vi "Pockels Cal_Update core.vi"(7 "Create new?":bool, 9 "New cal section (empty objectives removed)":string[][](array[string])=[["Cal Wavelength", "", "", "", "", "", ""], ["920", "", "", "", "", "", ""], ["Cal subset indexes", "", "", "", "", "", ""], ["0", "15", "", "", "", "", ""], ["Cal data", "", "", "", "", "", ""], ["Pockels V", "No objective", "Olympus 60X", "Empty new", "Olympus 20X", "Brand new", "Nikon 25X"], ["0", "11", "1", "", "1000", "100", ""], ["0.111", "22", "2", "", "2000", "200", ""], ["0.222", "33", "3", "", "3000", "300", ""], ["0.333", "44", "4", "", "", "400", ""], ["0.444", "55", "5", "", "", "500", ""], ["0.5", "66", "6", "", "", "", ""], ["0.6", "77", "7", "", "", "", ""], ["0.7", "88", "8", "", "", "", ""], ["0.8", "99", "9", "", "", "", ""], ["0.9", "00", "0", "", "", "", ""], ["1", "11", "1", "", "", "", ""], ["1.1", "22", "2", "", "", "", ""], ["1.2", "33", "3", "", "", "", ""], ["1.3", "44", "4", "", "", "", ""], ["1.4", "55", "5", "", "", "", ""], ["1.5", "66", "6", "", "", "", ""], ["1.6", "77", "7", "", "", "", ""], ["1.7", "88", "8", "", "", "", ""], ["1.8", "99", "9", "", "", "", ""], ["1.9", "00", "0", "", "", "", ""], ["2", "11", "1", "900", "9000", "", ""]], 11 "Loaded cal file":string[][](array[string])=[["Cal Wavelength", "", "", "", "", ""], ["800", "", "", "", "", ""], ["Cal subset indexes", "", "", "", "", ""], ["0", "15", "", "", "", ""], ["Cal data", "", "", "", "", ""], ["Pockels V", "No objective", "Olympus 20X", "Nikon 25X", "Olympus 40X", "Olympus 60X"], ["0", "1.9", "", "", "", ""], ["0.1", "3.7", "", "", "", ""], ["0.2", "8.2", "", "", "", ""], ["0.3", "15.4", "", "", "", ""], ["0.4", "24.5", "", "", "", ""], ["0.5", "35.5", "", "", "", ""], ["0.6", "47.8", "", "", "", ""], ["0.7", "61.3", "", "", "", ""], ["0.8", "73.4", "", "", "", ""], ["0.9", "90", "", "", "", ""], ["1", "104", "", "", "", ""], ["1.1", "116", "", "", "", ""], ["1.2", "128", "", "", "", ""], ["1.3", "138", "", "", "", ""], ["1.4", "148", "", "", "", ""], ["1.5", "154", "", "", "", ""], ["1.6", "157", "", "", "", ""], ["1.7", "155", "", "", "", ""], ["1.8", "154", "", "", "", ""], ["1.9", "154", "", "", "", ""], ["2", "154", "", "", "", ""], ["", "", "", "", "", ""], ["Cal Wavelength", "", "", "", "", ""], ["920", "", "", "", "", ""], ["Cal subset indexes", "", "", "", "", ""], ["0", "15", "", "", "", ""], ["Cal data", "", "", "", "", ""], ["Pockels V", "No objective", "Olympus 20X", "Nikon 25X", "Olympus 40X", "Olympus 60X"], ["0", "1.9", "1", "2", "", ""], ["0.1", "3.7", "1", "2", "", ""], ["0.2", "8.2", "1", "2", "", ""], ["0.3", "15.4", "1", "2", "", ""], ["0.4", "24.5", "1", "2", "", ""], ["0.5", "35.5", "1", "", "", ""], ["0.6", "47.8", "1", "", "", ""], ["0.7", "61.3", "1", "", "", ""], ["0.8", "73.4", "", "", "", ""], ["0.9", "90", "", "", "", ""], ["1", "104", "", "", "", ""], ["1.1", "116", "", "", "", ""], ["1.2", "128", "", "", "", ""], ["1.3", "138", "", "", "", ""], ["1.4", "148", "", "", "", ""], ["1.5", "154", "", "", "", ""], ["1.6", "157", "", "", "", ""], ["1.7", "155", "", "", "", ""], ["1.8", "154", "", "", "", ""], ["1.9", "154", "1", "2", "", ""], ["2", "154", "1", "2", "", ""], ["", "", "", "", "", ""]]) -> (2 "Cal file strings":string[][](array[string]))   [LabVIEW 2020]
panel:
  out "Current wavelength":dbl
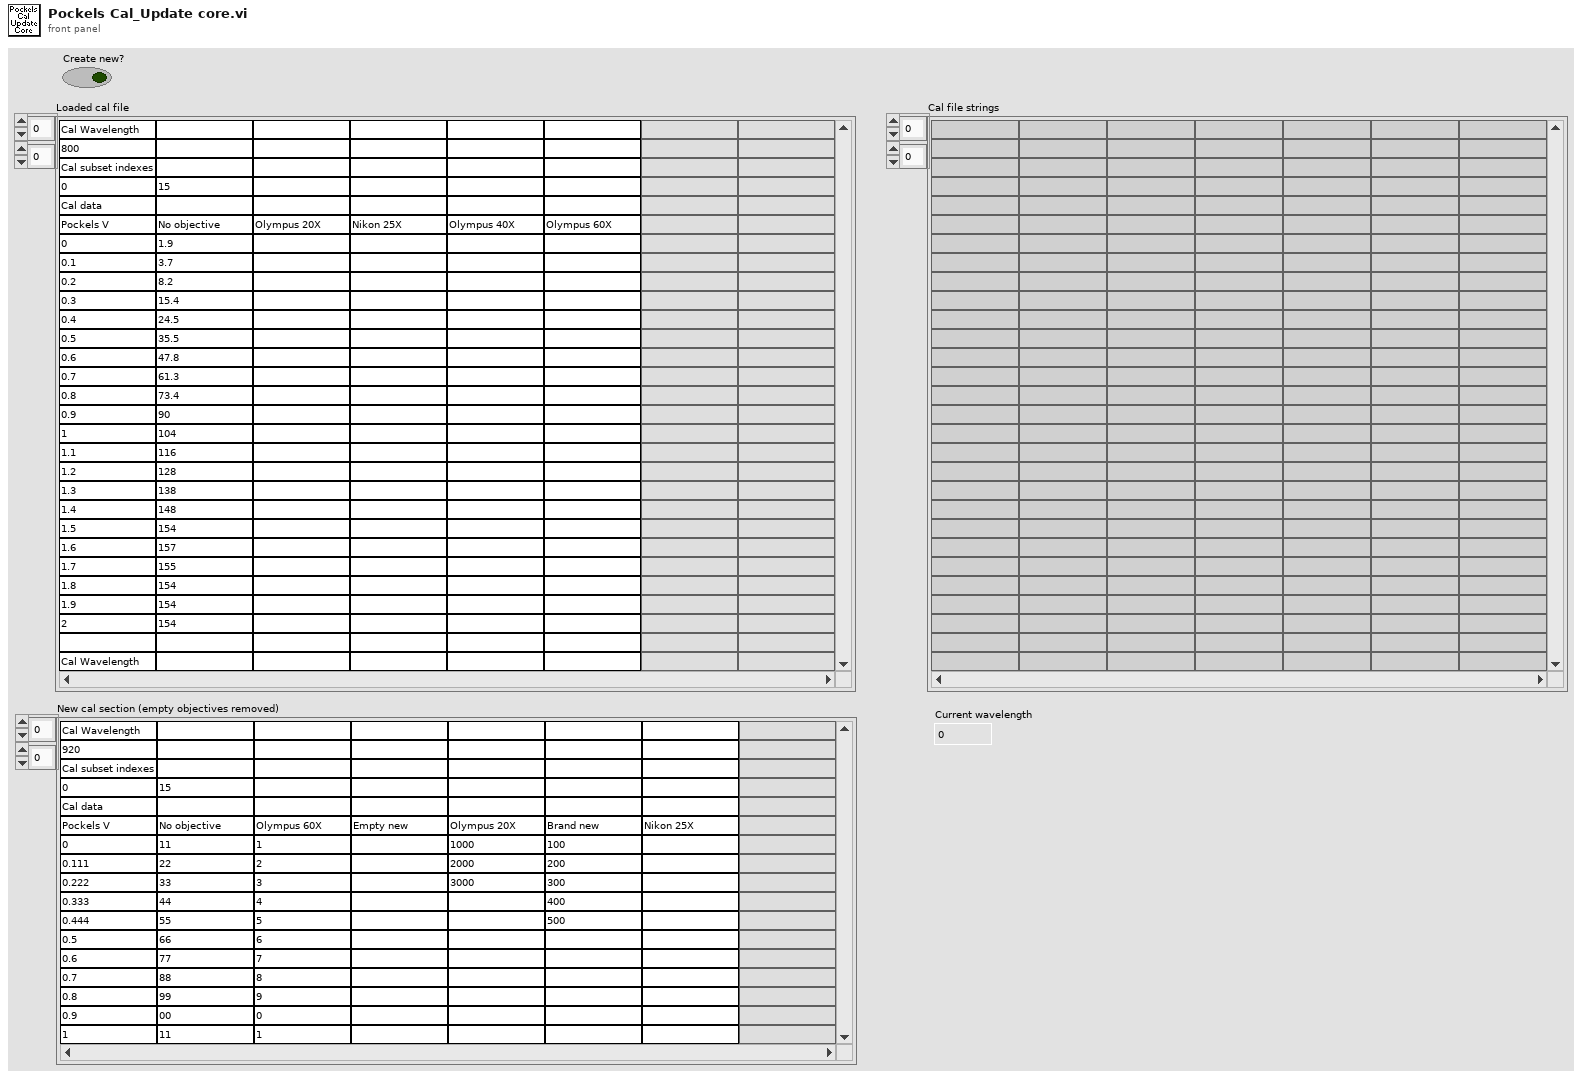
[diagram p1: front panel]
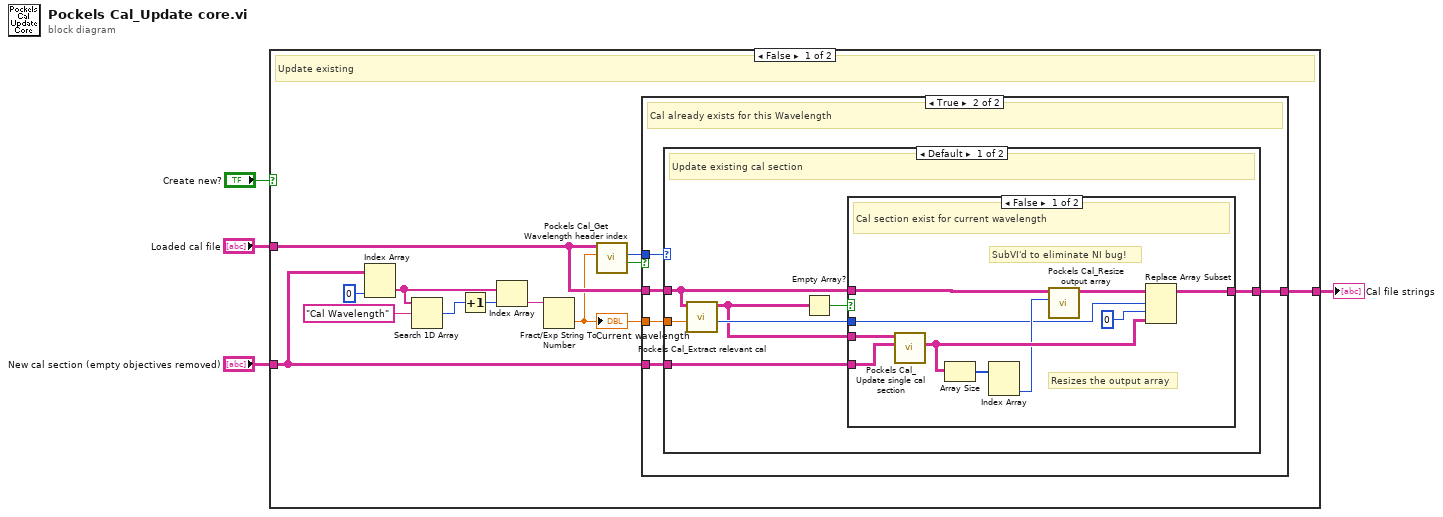
[diagram p0: block diagram]
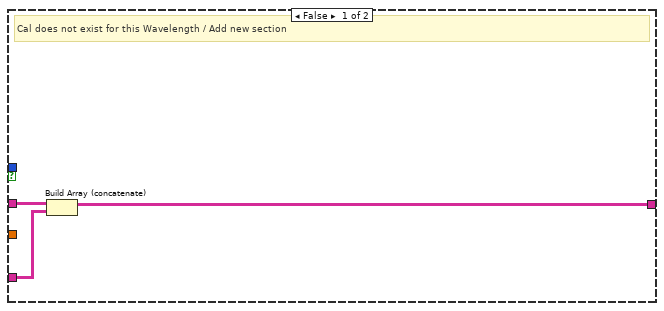
[diagram p2: hidden frame]
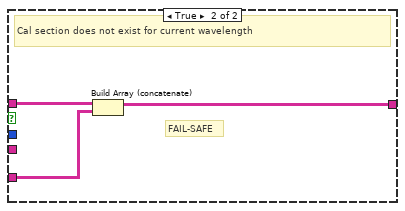
[diagram p3: hidden frame]
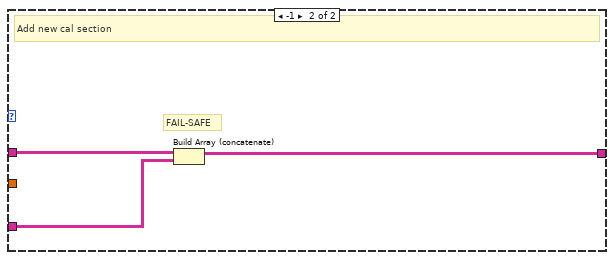
[diagram p4: hidden frame]
diagram:
  n1 = case shown="False" "Create new?" {
    tunnel: [w11 w48] -> w4
    tunnel: "Loaded cal file" -> [w7 _]
    tunnel: "New cal section (empty objectives removed)" -> [w6 w48]
    frame False {
      # "Update existing"
      n2 = Index Array(array=w6, index (col)=0 ("disabled index (col)")) -> (element=w14:string[])  [unwired: 1 in]
      n3 = Search 1D Array(1D array=w14, element="Cal Wavelength") -> (index of element=w15:i32)  [unwired: 1 in]
      n4 = Increment(x=w15) -> (x+1=w12:i32)
      n5 = Index Array(array=w14, index=w12) -> (element=w13:string)
      n6 = Fract/Exp String To Number(string=w13) -> (number=w5:dbl)  [unwired: 3 in, 1 out]
      "Current wavelength" <- w5
      n7 = call "Pockels Cal_Get Wavelength header index.vi"("Waveform"=w5, "Loaded cal file"=w7) -> ("Cal already exists for this wavelength?"=w9:bool, "Index of \"Cal Wavelength\" header"=w8:i32)  [unwired: 8 in]
      n8 = case shown="True" w9 {
        tunnel: w7 -> [w19 w24]
        tunnel: w6 -> [w18 w23]
        tunnel: [w17 w22] -> w11
        tunnel: w8 -> [_ w21]
        tunnel: w5 -> [_ w20]
        frame False {
          # "Cal does not exist for this Wavelength / Add new section"
          n9 = Build Array (concatenate)(w19, w18) -> (w17:string[][])
        }
        frame True {
          # "Cal already exists for this Wavelength"
          n10 = case shown="Default" w21 {
            tunnel: w24 -> [w30 w47]
            tunnel: w23 -> [w29 w45]
            tunnel: [w28 w46] -> w22
            tunnel: w20 -> [w25 _]
            frame Default {
              # "Update existing cal section"
              n11 = call "Pockels Cal_Extract relevant cal.vi"("Wavelength value"=w25, "Loaded table"=w30) -> ("Index of replacement"=w27:i32, "Relevant cal only"=w26:string[][])  [unwired: 6 in, 2 out]
              n12 = Empty Array?(array=w26) -> (empty?=w31:bool)
              n13 = case shown="False" w31 {
                tunnel: w30 -> [w34 w44]
                tunnel: w29 -> [w39 w42]
                tunnel: [w41 w43] -> w28
                tunnel: w27 -> [w32 _]
                tunnel: w26 -> [w40 _]
                frame False {
                  # "SubVI'd to eliminate NI bug!"
                  # "Resizes the output array"
                  # "Cal section exist for current wavelength"
                  n14 = call "Pockels Cal_Update single cal section.vi"("New cal section"=w39, "Loaded cal section"=w40) -> ("Updated cal section"=w36:string[][])  [unwired: 9 in]
                  n15 = Array Size(array=w36) -> (size(s)=w37:i32[])
                  n16 = Index Array(array=w37) -> (element #2=w35:i32)  [unwired: 2 in, 1 out]
                  n17 = call "Pockels Cal_Resize output array.vi"("Numeric"=w35, "Loaded cal file"=w34) -> ("Array"=w33:string[][])  [unwired: 9 in]
                  n18 = Replace Array Subset "Replace Array Subset"(array=w33, new element=w36, index (row)=w32, index (col)=0 ("disabled index (col)")) -> (w41:string[][])
                }
                frame True {
                  # "FAIL-SAFE"
                  # "Cal section does not exist for current wavelength"
                  n19 = Build Array (concatenate)(w44, w42) -> (w43:string[][])
                }
              }
            }
            frame -1 {
              # "FAIL-SAFE"
              # "Add new cal section"
              n20 = Build Array (concatenate)(w47, w45) -> (w46:string[][])
            }
          }
        }
      }
    }
    frame True {
      # "Create new file"
    }
  }
  "Cal file strings" <- w4
